vi "NISE.local.Write Session.TCPIP.KeepAliveTimeout.vi"(8 "error in (no error)":errorcluster, 10 "Session.TCPIP.KeepAliveTimeout":dbl, 11 "SLSC Local in":refnum<class "SLSC Interface.lvclass">) -> (0 "error out":errorcluster, 3 "SLSC Local out":refnum<class "SLSC Interface.lvclass">)   [LabVIEW 2016, in "SLSC Interface.lvclass"]
uses:
  SLSC Interface Class/SLSC Interface.lvclass
  SLSC Interface Class/NISE.Read session.vi
  <resource>/objmgr/slsc.rc
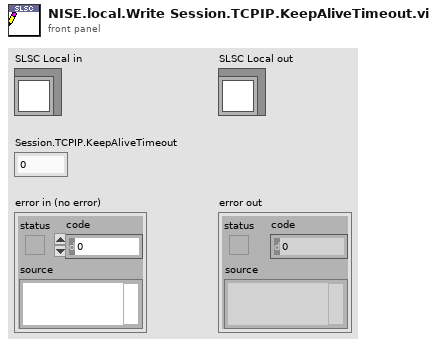
[diagram p1: front panel]
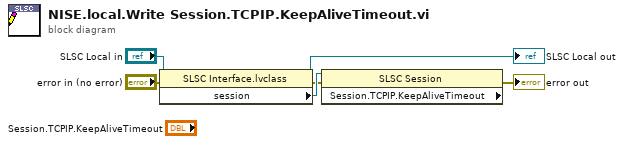
[diagram p0: block diagram]
diagram:
  n1 = property class="SLSC Interface.lvclass"(reference="SLSC Local in", error in="error in (no error)") -> (reference out=→"SLSC Local out":refnum<class "SLSC Interface.lvclass">, error out=w5:errorcluster, "session"=w6:refnum<k21>)
  n2 = property class="SLSC Session" props=["Session.TCPIP.KeepAliveTimeout"](reference=w6, error in=w5) -> (error out=→"error out":errorcluster)  [unwired: 2 out]
